vi "FormatErrorString.vi"(8 "error in (no error)":errorcluster) -> (2 "message":string=" INSTRUCTIONS:\r\rNormal Use:  When using subVIs that incorporate the error in/error out (or error I/O) structure, place this handler where you want to inform the user of an error, typically at the end of the I/O data path, as the last action of the program.  If the error in error? is ERROR, the handler creates a message describing the error and its source.  If the type of dialog = 1 (default), the message is displayed to the user, who can only acknowedge it.  If the type = 2, the user can acknowledge the message or abort execution; aborting a program with active I/O is not recommended.  If the type = 0, no message is displayed; this is used to process the error programmatically, and the error out cluster elements are wired to individual terminals for that reason.  \r\rOther Use:\n\r\nlocal testing.  To test the error code of a subVI or function that does not have the error I/O structure, you can wire its error code and a source string to the local error code and error source inputs.  If error in error? indicates no error and error code is not equal to 0, the local code and source are substituted for the error in values, and error? is set TRUE (ERROR).", 3 "Array":u32[][](array[numeric]))   [LabVIEW 2019, in "RT_Game.lvlib" / "Engine.lvclass"]
uses:
  Engine.lvclass
  <vilib>/Utility/error.llb/DialogType.ctl
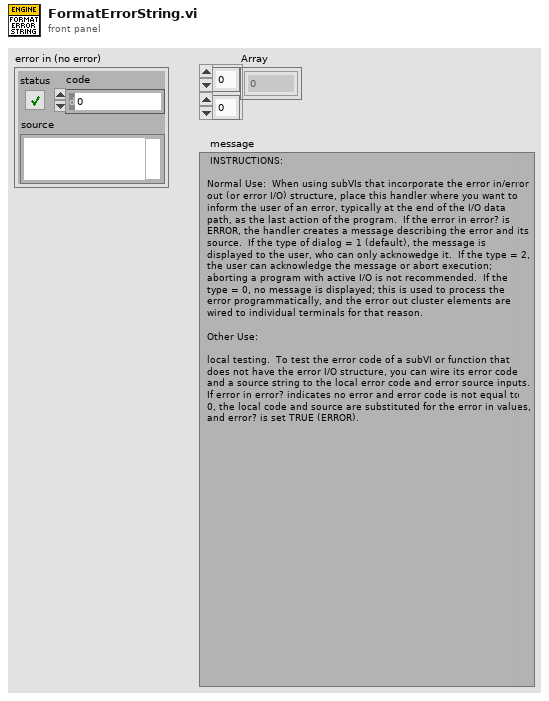
[diagram p1: front panel]
types:
  T1 = typedef "DialogType.ctl" = u16
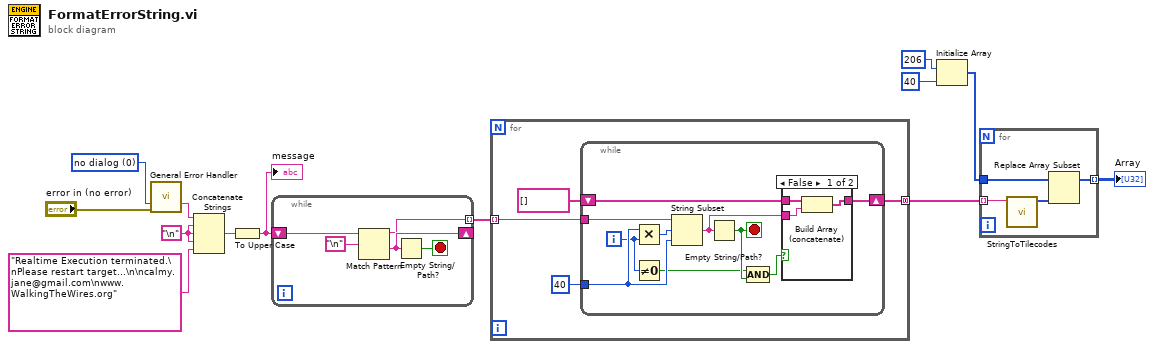
[diagram p0: block diagram]
diagram:
  w13 = "\n"
  w3 = T1 0 items=["no dialog", "OK message", "continue or stop message", "OK message + warnings", "continue/stop + warnings"] ("type of dialog (OK msg:1)")
  n1 = call <vilib>:"General Error Handler.vi"("type of dialog (OK msg:1)"=w3, "error in (no error)"="error in (no error)") -> ("message"=w8:string)  [unwired: 9 in, 4 out]
  n2 = Concatenate Strings(w8, w13, w13, w13, "Realtime Execution terminated.\nPlease restart target...\n\ncalmy.jane@gmail.com\nwww.WalkingTheWires.org" ("string")) -> (w11:string)
  n3 = To Upper Case(1:w11) -> (0:w10:string)
  "message" <- w10
  n4 = while {
    shift-right: [w15] -> _
    shift-left: w10 -> [w18]
    tunnel: [w14] -> w9 mode=indexing
    stop <- w16 stop-if-true
    n5 = Match Pattern(string=w18, regular expression="\n") -> (before substring=w14:string, after substring=w15:string)  [unwired: 1 in, 2 out]
    n6 = Empty String/Path?(string/path=w15) -> (empty?=w16:bool)
  }
  n7 = for {
    tunnel: [w20] -> w2 mode=concatenating
    tunnel: w9 -> [w19] mode=indexing
    n8 = while {
      tunnel: w19 -> [w32]
      tunnel: 40 -> [w30]
      shift-right: [w28] -> w20
      shift-left: string[] [] ("before substring") -> [w29]
      i -> [w24]
      stop <- w26 stop-if-true
      n9 = Multiply(x=w30, y=w24) -> (x*y=w31:i32)
      n10 = Not Equal To 0?(x=w24) -> (x != 0?=w23:bool)
      n11 = String Subset(string=w32, offset (0)=w31, length (rest)=w30) -> (substring=w27:string)
      n12 = Empty String/Path?(string/path=w27) -> (empty?=w26:bool)
      n13 = Compound Arithmetic op=AND(w23, w26) -> (w25:bool)
      n14 = case shown="False" w25 {
        tunnel: w29 -> [w35 w36]
        tunnel: [w34 w36] -> w28
        tunnel: w27 -> [w33 _]
        frame False {
          n15 = Build Array (concatenate)(w35, w33) -> (w34:string[])
        }
        frame True {
        }
      }
    }
  }
  n16 = Initialize Array(u32 206, 40 ("dimension size")) -> (w7:u32[])
  n17 = for {
    tunnel: [w37] -> w1 mode=indexing
    tunnel: w2 -> [w39] mode=indexing
    tunnel: w7 -> [w40]
    n18 = call "StringToTilecodes.vi"("String"=w39) -> ("Tilecodes"=w38:u32[])  [unwired: 10 in]
    n19 = Replace Array Subset(array=w40, new element=w38) -> (w37:u32[])  [unwired: 1 in]
  }
  "Array" <- w1
